vi "error_monitor.vi"(8 "error in (no error)":errorcluster caption="エラー入力（エラーなし）", 11 "エラー情報":cluster{"キュー名":string, "コマンド名":string}) -> (0 "error out":errorcluster caption="エラー出力")   [LabVIEW 2015]
uses:
  error_handler_command.ctl
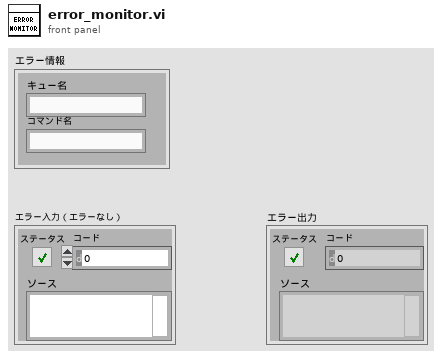
[diagram p1: front panel]
types:
  T1 = typedef "error_handler_command.ctl" = enum16{"reset", "get", "set"}
  T2 = enum16{"open", "replace", "create", "open or create", "replace or create", "replace or create with confirmation"}
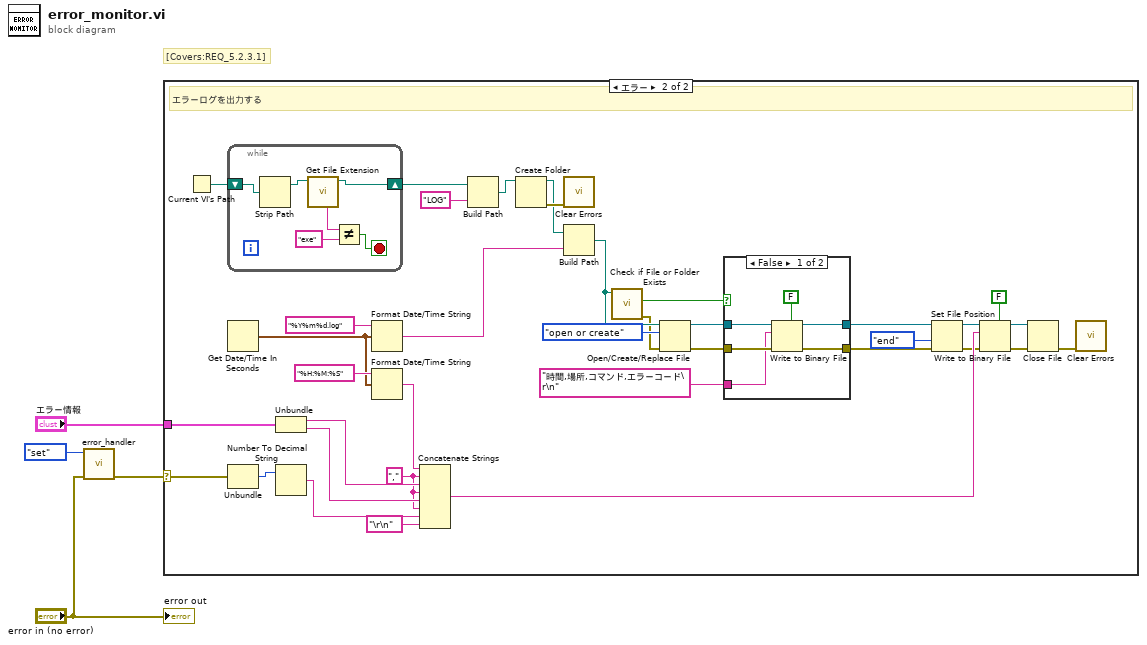
[diagram p0: block diagram]
diagram:
  # "[Covers:REQ_5.2.3.1]"
  n1 = call "error_handler.vi"("error in (no error)"="error in (no error)", "command"=error_handler_command."set") -> ("error out"=w1:errorcluster)  [unwired: 8 in, 1 out]
  n2 = case "ケースストラクチャ" shown="エラー" w1 {
    selector: w1 -> [_ w29]
    tunnel: "エラー情報" -> [_ w18]
    frame No Error {
    }
    frame Error {
      w15 = "," ("文字列")
      # "エラーログを出力する"
      n3 = Current VI's Path ("現在のVIのパス")() -> (path=w40:path)
      n4 = while "Whileループ" {
        shift-right: [w41] -> w39
        shift-left: w40 -> [w46]
        stop <- w42 stop-if-true
        n5 = Strip Path ("パスをストリップ")(path=w46) -> (stripped path=w45:path)  [unwired: 1 out]
        n6 = call <vilib>:"Get File Extension.vi"("file"=w45) -> ("dup file"=w41:path, "unmodified file extension"=w44:string)  [unwired: 6 in, 3 out]
        n7 = Not Equal? ("等しくない?")(x=w44, y="exe") -> (x != y?=w42:bool)
      }
      n8 = Get Date/Time In Seconds ("日付/時間を秒で取得")() -> (seconds since 1Jan1904=w27:timestamp)
      n9 = Unbundle ("バンドル解除")(w29) -> ("code"=w25:i32)  [unwired: 2 out]
      n10 = Unbundle ("バンドル解除")(w18) -> ("キュー名"=w16:string, "コマンド名"=w17:string)
      n11 = Number To Decimal String ("数値を10進数文字列に変換")(number=w25) -> (decimal integer string=w24:string)  [unwired: 1 in]
      n12 = Format Date/Time String ("日付/時間文字列をフォーマット")(time format string (%c)="%Y%m%d.log" ("時間形式文字列（%c）"), seconds (now)=w27) -> (date/time string=w32:string)  [unwired: 1 in]
      n13 = Format Date/Time String ("日付/時間文字列をフォーマット")(time format string (%c)="%H:%M:%S" ("時間形式文字列（%c）"), seconds (now)=w27) -> (date/time string=w26:string)  [unwired: 1 in]
      n14 = Concatenate Strings ("文字列連結")(w26, w15, w16, w15, w17, w15, w24, "\r\n" ("文字列")) -> (w22:string)
      n15 = Build Path ("パス作成")(base path=w39, name or relative path="LOG" ("名前または相対パス")) -> (appended path=w37:path)
      n16 = Create Folder ("フォルダを作成")(path (use dialog)=w37) -> (created path=w34:path, error out=w36:errorcluster)  [unwired: 2 in, 1 out]
      n17 = call <vilib>:"Clear Errors.vi"("error in (no error)"=w36) -> ()  [unwired: 5 in, 2 out]
      n18 = Build Path ("パス作成")(base path=w34, name or relative path=w32) -> (appended path=w13:path)
      n19 = call <vilib>:"Check if File or Folder Exists.vi"("path"=w13) -> ("error out"=w6:errorcluster, "file or folder exists?"=w8:bool)  [unwired: 8 in, 1 out]
      n20 = Open/Create/Replace File ("ファイルを開く/作成/置換")(file path (use dialog)=w13, error in=w6, operation (0:open)=T2."open or create" ("操作（0:open）")) -> (refnum out=w10:refnum<file>, error out=w9:errorcluster)  [unwired: 3 in, 1 out]
      n21 = case "ケースストラクチャ" shown="FALSE" w8 {
        tunnel: [w52 w54] -> w12
        tunnel: [w51 w53] -> w11
        tunnel: w10 -> [w50 w54]
        tunnel: w9 -> [w49 w53]
        tunnel: "時間,場所,コマンド,エラーコード\r\n" ("時間形式文字列（%c）") -> [w48 _]
        frame False {
          n22 = Write to Binary File ("バイナリファイルに書き込む")(file (use dialog)=w50, data=w48, error in=w49, 5:FALSE ("配列または文字列サイズを先頭に追加?(T)")) -> (refnum out=w52:refnum<file>, error out=w51:errorcluster)  [unwired: 2 in, 1 out]
        }
        frame True {
        }
      }
      n23 = Set File Position ("ファイル位置を設定")(refnum=w12, from (0:start)=enum16{"start", "end", "current"}."end" ("基点（0:start）"), error in=w11) -> (refnum out=w21:refnum<file>, error out=w20:errorcluster)  [unwired: 1 in]
      n24 = Write to Binary File ("バイナリファイルに書き込む")(file (use dialog)=w21, data=w22, error in=w20, 5:FALSE ("配列または文字列サイズを先頭に追加?(T)")) -> (refnum out=w30:refnum<file>, error out=w31:errorcluster)  [unwired: 2 in, 1 out]
      n25 = Close File ("ファイルを閉じる")(refnum=w30, error in=w31) -> (error out=w14:errorcluster)  [unwired: 1 out]
      n26 = call <vilib>:"Clear Errors.vi"("error in (no error)"=w14) -> ()  [unwired: 5 in, 2 out]
    }
  }
  "error out" <- "error in (no error)"
